vi "180 deg rot.vi"(1 "x (deg)":dbl) -> (0 "x rot 180":dbl)   [LabVIEW 2019]
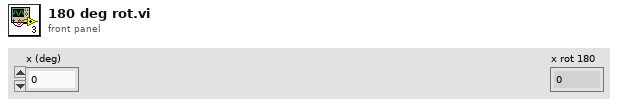
[diagram p1: front panel]
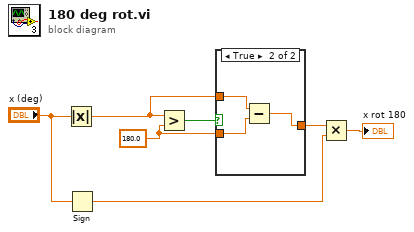
[diagram p0: block diagram]
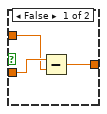
[diagram p2: hidden frame]
diagram:
  w6 = 180.0
  n1 = Absolute Value(x="x (deg)") -> (abs(x)=w5:dbl)
  n2 = Sign(1:"x (deg)") -> (0:w2:dbl)
  n3 = Greater?(x=w5, y=w6) -> (0:w7:bool)
  n4 = case shown="True" w7 {
    tunnel: w6 -> [w10 w12]
    tunnel: w5 -> [w9 w13]
    tunnel: [w8 w11] -> w4
    frame False {
      n5 = Subtract(x=w10, y=w9) -> (x-y=w8:dbl)
    }
    frame True {
      n6 = Subtract(x=w13, y=w12) -> (x-y=w11:dbl)
    }
  }
  n7 = Multiply(x=w4, y=w2) -> (x*y=→"x rot 180":dbl)
